vi "Autonomous Independent.vi"   [LabVIEW 2014]
doc: "This VI is called when autonomous begins, and will automatically be terminated when autonomous ends. You can carry out timed or sensor driven robot movement independently without needing to return to the caller."
uses:
  <vilib>/Rock Robotics/SystemInterfaces/i2clib/i2c_bus.ctl
  <vilib>/Rock Robotics/Network Tables/SD Read Number.vi
  <vilib>/Rock Robotics/WPI/RobotDrive/WPI_RobotDriveGetSetRefNum.vi
  <vilib>/Rock Robotics/WPI/RobotDrive/WPI_RobotDriveMecanumDrive_Cartesian.vi
  Robot Global Data.vi
panel:
  # "Be sure to right-click and choose Data Operations>>Make Current Value default if you want to save the array values with the VI"
types:
  T1 = typedef "WPI_RobotDriveDevRef.ctl" = cluster{"DevStatus":errorcluster, "Motors[]":T2[], "Square Inputs":bool, "Max Output":dbl}
  T2 = typedef "WPI_MotorControlDeviceRef.ctl" = cluster{"DeviceStatus":errorcluster, "Type":T3, "PWM":cluster{"Controller":T4, "PWM Channel":T5, "DeadBand":T6}, "CAN":cluster{"Device Number":u8, "Control Mode":T7, "Semaphore":T8, "Max Vout":dbl, "TalonSRX Control Mode":T9}, "Invert":bool, "TransformRef":T10, "InvTransformRef":T10}
  T3 = typedef "WPI_MotorControlType.ctl" = enum16{"PWM", "CAN", "CANTalonSRX"}
  T4 = typedef "FPGA_TypedefDigitalModule.ctl" = enum16{"Controller 1"}
  T5 = typedef "FPGA_DIOPWMChannel.ctl" = enum8{"PWM 0", "PWM 1", "PWM 2", "PWM 3", "PWM 4", "PWM 5", "PWM 6", "PWM 7", "PWM 8", "PWM 9", "PWM MXP 0", "PWM MXP 1", "PWM MXP 2", "PWM MXP 3", "PWM MXP 4", "PWM MXP 5", "PWM MXP 6", "PWM MXP 7", "PWM MXP 8", "PWM MXP 9", "Invalid"}
  T6 = typedef "WPI_PWMDeadband.ctl" = cluster{"Name":string, "maxPositivePwm":i32, "minPositivePwm":i32, "centerPwm":i32, "maxNegativePwm":i32, "minNegativePwm":i32, "angularRange":u16}
  T7 = typedef "WPI_CANJaguar_ControlMode.ctl" = enum8{"Percent VBus", "Current", "Speed", "Position", "Voltage"}
  T8 = typedef "Semaphore RefNum" = refnum<k1>
  T9 = typedef "WPI_CANTalonSRX_APIControlMode.ctl" = enum8{"Percent VBus", "Speed", "Position", "Slave", "Unchanged / Invalid"}
  T10 = typedef "WPI_PWMTransform_ConPane.ctl" = refnum<vi>
  T11 = typedef "WPI_EncoderDevRef.ctl" = cluster{"DevStatus":errorcluster, "EncoderIndex":T12, "CounterIndex":T13, "DistancePerCount":dbl, "Decoding Type":T14}
  T12 = typedef "FPGA_EncoderIdx.ctl" = enum8{"Enc 0", "Enc 1", "Enc 2", "Enc 3", "Enc 4", "Enc 5", "Enc 6", "Enc 7", "Invalid"}
  T13 = typedef "FPGA_CounterCtrSystemIndex.ctl" = enum8{"Ctr 0", "Ctr 1", "Ctr 2", "Ctr 3", "Ctr 4", "Ctr 5", "Ctr 6", "Ctr 7", "Invalid"}
  T14 = typedef "WPI_EncoderType.ctl" = enum16{"1x", "2x", "4x"}
  T15 = typedef "WPI_GyroDevRef.ctl" = cluster{"DevStatus":errorcluster, "Analog Module":T16, "Analog Channel":T17, "Offset":dbl, "Gain (VoltsPerDegree/Second)":dbl}
  T16 = typedef "FPGA_TypedefAnalogModule.ctl" = enum16{"Controller 1"}
  T17 = typedef "FPGA_AIChannel.ctl" = enum8{"AI 0", "AI 1", "AI 2", "AI 3", "AI MXP 0", "AI MXP 1", "AI MXP 2", "AI MXP 3", "Invalid"}
  T18 = typedef "WPI_I2CDevRef.ctl" = cluster{"DevStatus":errorcluster, "Controller":T4, "Device Address":u8, "Handle":i32, "I2C Bus":T19}
  T19 = typedef "i2c_bus.ctl" = enum16{"I2C On-Board", "I2C MXP", "Invalid"}
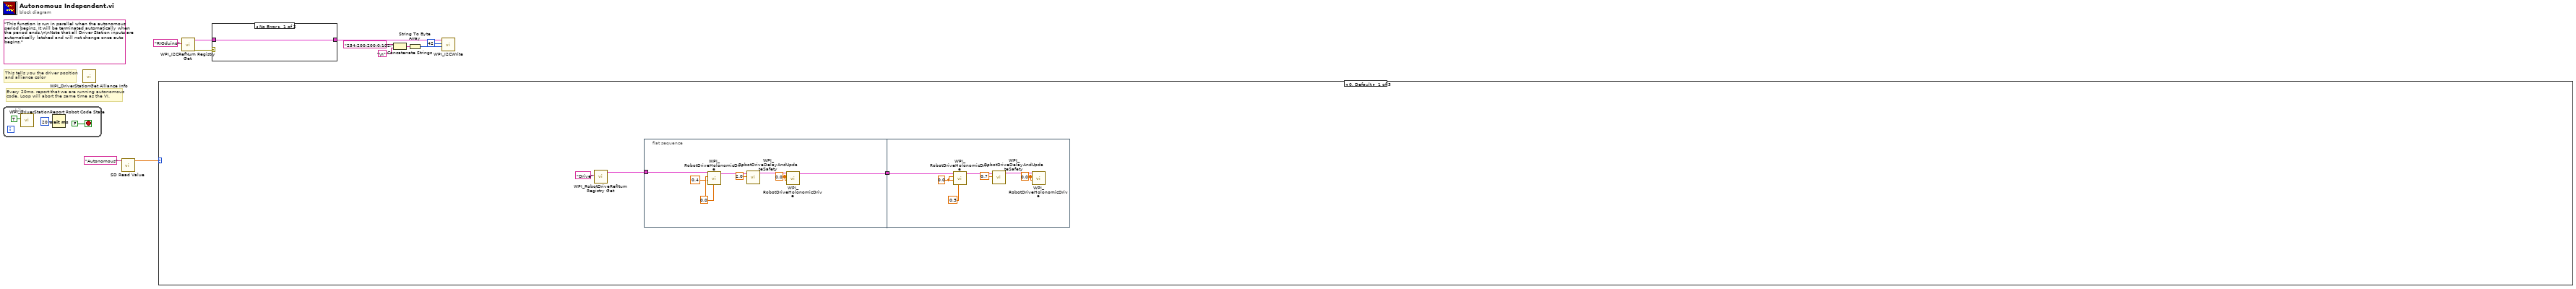
[diagram p0: block diagram]
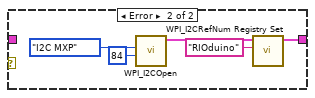
[diagram p2: hidden frame]
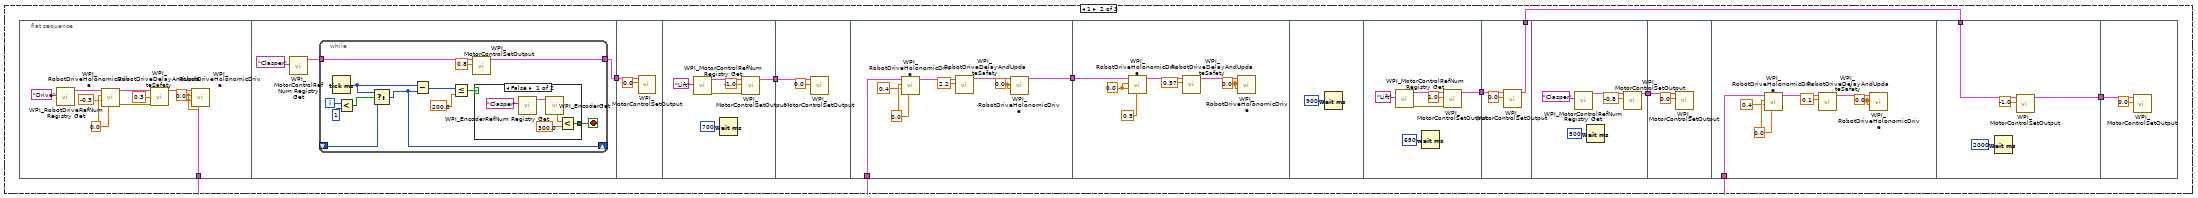
[diagram p3: hidden frame]
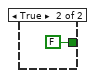
[diagram p4: hidden frame]
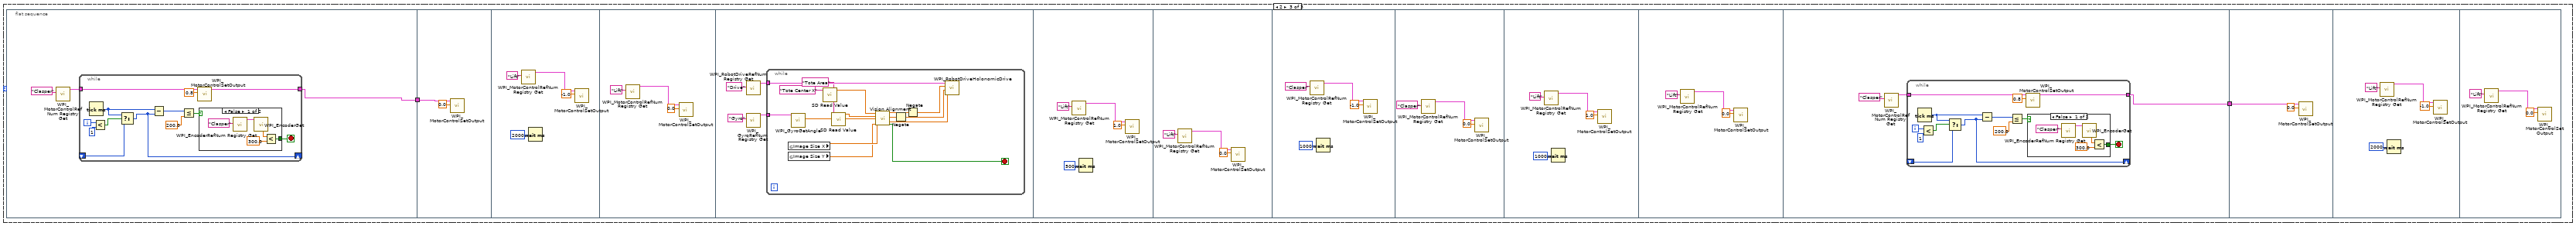
[diagram p5: hidden frame]
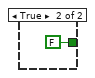
[diagram p6: hidden frame]
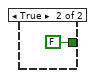
[diagram p7: hidden frame]
diagram:
  (unwired) "This function is run in parallel when the autonomous period begins. It will be terminated automatically when the period ends.\n\nNote that all Driver Station inputs are automatically latched and will not change once auto begins."
  # "Every 20ms, report that we are running autonomous\ncode. Loop will abort the same time as the VI."
  # "This tells you the driver position\nand alliance color"
  n1 = while {
    stop <- FALSE stop-if-true
    n2 = call <vilib>:"WPI_DriverStationReport Robot Code State.vi"("Autonomous"=TRUE) -> ()  [unwired: 10 in, 1 out]
    n3 = Wait (ms)(milliseconds to wait=u32 20) -> ()  [unwired: 1 out]
  }
  n4 = call <vilib>:"WPI_DriverStationGet Alliance Info.vi"() -> ()  [unwired: 12 out]
  n5 = call-poly <vilib>:"SD Read Value.vi"("Name"="Autonomous") -> ("Numeric"=w10:dbl)  [unwired: 8 in, 2 out]
  n6 = case shown="0, Default" w10 {
    frame 0, Default {
      n7 = call <vilib>:"WPI_RobotDriveRefNum Registry Get.vi"("refnum name"="Drive") -> ("RobotDriveDevRef"=w15:T1)  [unwired: 9 in, 1 out]
      n8 = flat-sequence {
        tunnel: [w19] -> w17
        tunnel: w15 -> [w18]
        tunnel: w17 -> [w26]
        frame #0 {
          w21 = 0.0
          w22 = 0.0 ("X")
          n9 = call-poly <vilib>:"WPI_RobotDriveHolonomicDrive.vi"("Rotation"=w21, "Y"=0.4 ("X"), "X"=w21, "RobotDriveDevRef"=w18) -> ("RobotDriveDevRef"=w25:T1)  [unwired: 5 in, 2 out]
          n10 = call <vilib>:"WPI_RobotDriveDelayAndUpdateSafety.vi"("Delay (s)"=2.0, "RobotDriveDevRef"=w25) -> ("RobotDriveDevRef 2"=w23:T1)  [unwired: 8 in, 1 out]
          n11 = call-poly <vilib>:"WPI_RobotDriveHolonomicDrive.vi"("Rotation"=w22, "Y"=w22, "X"=w22, "RobotDriveDevRef"=w23) -> ("RobotDriveDevRef"=w19:T1)  [unwired: 5 in, 2 out]
        }
        frame #1 {
          w30 = 0.0 ("X")
          w32 = 0.0 ("X")
          n12 = call-poly <vilib>:"WPI_RobotDriveHolonomicDrive.vi"("Rotation"=0.5, "Y"=w32, "X"=w32, "RobotDriveDevRef"=w26) -> ("RobotDriveDevRef"=w27:T1)  [unwired: 5 in, 2 out]
          n13 = call <vilib>:"WPI_RobotDriveDelayAndUpdateSafety.vi"("Delay (s)"=0.7, "RobotDriveDevRef"=w27) -> ("RobotDriveDevRef 2"=w29:T1)  [unwired: 8 in, 1 out]
          n14 = call-poly <vilib>:"WPI_RobotDriveHolonomicDrive.vi"("Rotation"=w30, "Y"=w30, "X"=w30, "RobotDriveDevRef"=w29) -> ()  [unwired: 5 in, 3 out]
        }
      }
    }
    frame 1 {
      n15 = flat-sequence {
        tunnel: [w44] -> w36
        tunnel: [w51] -> w40
        tunnel: w40 -> [w74]
        tunnel: [w75] -> w39
        tunnel: w39 -> [w82]
        tunnel: w36 -> [w89]
        tunnel: [w83] -> w35
        tunnel: w35 -> [w92]
        tunnel: [w99] -> w38
        tunnel: w38 -> [w106]
        tunnel: [w105] -> w33
        tunnel: [w108] -> w37
        tunnel: w37 -> [w113]
        tunnel: w36 -> [w115]
        tunnel: [w123] -> w34
        tunnel: w33 -> [w122]
        tunnel: w34 -> [w126]
        frame #0 {
          w42 = 0.0
          w43 = 0.0 ("X")
          n16 = call <vilib>:"WPI_RobotDriveRefNum Registry Get.vi"("refnum name"="Drive") -> ("RobotDriveDevRef"=w50:T1)  [unwired: 9 in, 1 out]
          n17 = call-poly <vilib>:"WPI_RobotDriveHolonomicDrive.vi"("Rotation"=w42, "Y"=-0.3 ("X"), "X"=w42, "RobotDriveDevRef"=w50) -> ("error out"=w48:errorcluster, "RobotDriveDevRef"=w47:T1)  [unwired: 5 in, 1 out]
          n18 = call <vilib>:"WPI_RobotDriveDelayAndUpdateSafety.vi"("error in (no error)"=w48, "Delay (s)"=0.3, "RobotDriveDevRef"=w47) -> ("RobotDriveDevRef 2"=w45:T1)  [unwired: 7 in, 1 out]
          n19 = call-poly <vilib>:"WPI_RobotDriveHolonomicDrive.vi"("Rotation"=w43, "Y"=w43, "X"=w43, "RobotDriveDevRef"=w45) -> ("RobotDriveDevRef"=w44:T1)  [unwired: 5 in, 2 out]
        }
        frame #1 {
          n20 = call <vilib>:"WPI_MotorControlRefNum Registry Get.vi"("refnum name"="Clasper") -> ("MotorControlDevRef"=w52:T2)  [unwired: 9 in, 1 out]
          n21 = while {
            tunnel: w52 -> [w66]
            tunnel: [w64] -> w51
            shift-right: [w58] -> _
            shift-left: _ -> [w59]
            i -> [w57]
            stop <- w60 stop-if-true
            n22 = Tick Count (ms)() -> (millisecond timer value=w63:u32)
            n23 = Less?(x=w57, y=1) -> (x < y?=w55:bool)
            n24 = Select(t=w63, s=w55, f=w59) -> (s? t:f=w58:u32)
            n25 = Subtract(x=w63, y=w58) -> (x-y=w62:u32)
            n26 = Less Or Equal?(x=w62, y=200.0) -> (x <= y?=w61:bool)
            n27 = call <vilib>:"WPI_MotorControlSetOutput.vi"("Output"=0.8, "MotorControlDevRef"=w66) -> ("MotorControlDevRef"=w64:T2)  [unwired: 7 in, 2 out]
            n28 = case shown="False" w61 {
              tunnel: [w67 FALSE] -> w60
              frame False {
                n29 = call <vilib>:"WPI_EncoderRefNum Registry Get.vi"("refnum name"="Clasper") -> ("EncoderDevRef"=w71:T11)  [unwired: 9 in, 1 out]
                n30 = call <vilib>:"WPI_EncoderGet.vi"("EncoderDevRef"=w71) -> ("Rate"=w68:dbl)  [unwired: 5 in, 5 out]
                n31 = Less?(x=w68, y=300.0) -> (x < y?=w67:bool)
              }
              frame True {
              }
            }
          }
        }
        frame #2 {
          n32 = call <vilib>:"WPI_MotorControlSetOutput.vi"("Output"=0.0, "MotorControlDevRef"=w74) -> ()  [unwired: 7 in, 3 out]
        }
        frame #3 {
          n33 = call <vilib>:"WPI_MotorControlRefNum Registry Get.vi"("refnum name"="Lift") -> ("error out"=w79:errorcluster, "MotorControlDevRef"=w78:T2)  [unwired: 9 in]
          n34 = Wait (ms)(milliseconds to wait=u32 700) -> ()  [unwired: 1 out]
          n35 = call <vilib>:"WPI_MotorControlSetOutput.vi"("error in (no error)"=w79, "Output"=-1.0, "MotorControlDevRef"=w78) -> ("MotorControlDevRef"=w75:T2)  [unwired: 6 in, 2 out]
        }
        frame #4 {
          n36 = call <vilib>:"WPI_MotorControlSetOutput.vi"("Output"=0.0, "MotorControlDevRef"=w82) -> ()  [unwired: 7 in, 3 out]
        }
        frame #5 {
          w85 = 0.0
          w86 = 0.0 ("X")
          n37 = call-poly <vilib>:"WPI_RobotDriveHolonomicDrive.vi"("Rotation"=w85, "Y"=0.4 ("X"), "X"=w85, "RobotDriveDevRef"=w89) -> ("RobotDriveDevRef"=w90:T1)  [unwired: 5 in, 2 out]
          n38 = call <vilib>:"WPI_RobotDriveDelayAndUpdateSafety.vi"("Delay (s)"=2.2, "RobotDriveDevRef"=w90) -> ("RobotDriveDevRef 2"=w87:T1)  [unwired: 8 in, 1 out]
          n39 = call-poly <vilib>:"WPI_RobotDriveHolonomicDrive.vi"("Rotation"=w86, "Y"=w86, "X"=w86, "RobotDriveDevRef"=w87) -> ("RobotDriveDevRef"=w83:T1)  [unwired: 5 in, 2 out]
        }
        frame #6 {
          w94 = 0.0 ("X")
          w91 = 0.0 ("X")
          n40 = call-poly <vilib>:"WPI_RobotDriveHolonomicDrive.vi"("Rotation"=0.5, "Y"=w91, "X"=w91, "RobotDriveDevRef"=w92) -> ("RobotDriveDevRef"=w97:T1)  [unwired: 5 in, 2 out]
          n41 = call <vilib>:"WPI_RobotDriveDelayAndUpdateSafety.vi"("Delay (s)"=0.57, "RobotDriveDevRef"=w97) -> ("RobotDriveDevRef 2"=w95:T1)  [unwired: 8 in, 1 out]
          n42 = call-poly <vilib>:"WPI_RobotDriveHolonomicDrive.vi"("Rotation"=w94, "Y"=w94, "X"=w94, "RobotDriveDevRef"=w95) -> ()  [unwired: 5 in, 3 out]
        }
        frame #7 {
          n43 = Wait (ms)(milliseconds to wait=u32 900) -> ()  [unwired: 1 out]
        }
        frame #8 {
          n44 = call <vilib>:"WPI_MotorControlRefNum Registry Get.vi"("refnum name"="Lift") -> ("error out"=w103:errorcluster, "MotorControlDevRef"=w102:T2)  [unwired: 9 in]
          n45 = Wait (ms)(milliseconds to wait=u32 650) -> ()  [unwired: 1 out]
          n46 = call <vilib>:"WPI_MotorControlSetOutput.vi"("error in (no error)"=w103, "Output"=1.0, "MotorControlDevRef"=w102) -> ("MotorControlDevRef"=w99:T2)  [unwired: 6 in, 2 out]
        }
        frame #9 {
          n47 = call <vilib>:"WPI_MotorControlSetOutput.vi"("Output"=0.0, "MotorControlDevRef"=w106) -> ("MotorControlDevRef"=w105:T2)  [unwired: 7 in, 2 out]
        }
        frame #10 {
          n48 = call <vilib>:"WPI_MotorControlRefNum Registry Get.vi"("refnum name"="Clasper") -> ("MotorControlDevRef"=w110:T2)  [unwired: 9 in, 1 out]
          n49 = Wait (ms)(milliseconds to wait=u32 500) -> ()  [unwired: 1 out]
          n50 = call <vilib>:"WPI_MotorControlSetOutput.vi"("Output"=-0.8, "MotorControlDevRef"=w110) -> ("MotorControlDevRef"=w108:T2)  [unwired: 7 in, 2 out]
        }
        frame #11 {
          n51 = call <vilib>:"WPI_MotorControlSetOutput.vi"("Output"=0.0, "MotorControlDevRef"=w113) -> ()  [unwired: 7 in, 3 out]
        }
        frame #12 {
          w117 = 0.0
          w118 = 0.0 ("X")
          n52 = call-poly <vilib>:"WPI_RobotDriveHolonomicDrive.vi"("Rotation"=w117, "Y"=0.4 ("X"), "X"=w117, "RobotDriveDevRef"=w115) -> ("RobotDriveDevRef"=w121:T1)  [unwired: 5 in, 2 out]
          n53 = call <vilib>:"WPI_RobotDriveDelayAndUpdateSafety.vi"("Delay (s)"=0.1, "RobotDriveDevRef"=w121) -> ("RobotDriveDevRef 2"=w119:T1)  [unwired: 8 in, 1 out]
          n54 = call-poly <vilib>:"WPI_RobotDriveHolonomicDrive.vi"("Rotation"=w118, "Y"=w118, "X"=w118, "RobotDriveDevRef"=w119) -> ()  [unwired: 5 in, 3 out]
        }
        frame #13 {
          n55 = Wait (ms)(milliseconds to wait=u32 2000) -> ()  [unwired: 1 out]
          n56 = call <vilib>:"WPI_MotorControlSetOutput.vi"("Output"=-1.0, "MotorControlDevRef"=w122) -> ("MotorControlDevRef"=w123:T2)  [unwired: 7 in, 2 out]
        }
        frame #14 {
          n57 = call <vilib>:"WPI_MotorControlSetOutput.vi"("Output"=0.0, "MotorControlDevRef"=w126) -> ()  [unwired: 7 in, 3 out]
        }
      }
    }
    frame 2 {
      n58 = flat-sequence {
        tunnel: [w130] -> w128
        tunnel: w128 -> [w152]
        tunnel: [w203] -> w129
        tunnel: w129 -> [w224]
        frame #0 {
          n59 = call <vilib>:"WPI_MotorControlRefNum Registry Get.vi"("refnum name"="Clasper") -> ("MotorControlDevRef"=w131:T2)  [unwired: 9 in, 1 out]
          n60 = while {
            tunnel: w131 -> [w145]
            tunnel: [w143] -> w130
            shift-right: [w137] -> _
            shift-left: _ -> [w138]
            i -> [w136]
            stop <- w139 stop-if-true
            n61 = Tick Count (ms)() -> (millisecond timer value=w142:u32)
            n62 = Less?(x=w136, y=1) -> (x < y?=w134:bool)
            n63 = Select(t=w142, s=w134, f=w138) -> (s? t:f=w137:u32)
            n64 = Subtract(x=w142, y=w137) -> (x-y=w141:u32)
            n65 = Less Or Equal?(x=w141, y=200.0) -> (x <= y?=w140:bool)
            n66 = call <vilib>:"WPI_MotorControlSetOutput.vi"("Output"=0.8, "MotorControlDevRef"=w145) -> ("MotorControlDevRef"=w143:T2)  [unwired: 7 in, 2 out]
            n67 = case shown="False" w140 {
              tunnel: [w146 FALSE] -> w139
              frame False {
                n68 = call <vilib>:"WPI_EncoderRefNum Registry Get.vi"("refnum name"="Clasper") -> ("EncoderDevRef"=w150:T11)  [unwired: 9 in, 1 out]
                n69 = call <vilib>:"WPI_EncoderGet.vi"("EncoderDevRef"=w150) -> ("Rate"=w147:dbl)  [unwired: 5 in, 5 out]
                n70 = Less?(x=w147, y=300.0) -> (x < y?=w146:bool)
              }
              frame True {
              }
            }
          }
        }
        frame #1 {
          n71 = call <vilib>:"WPI_MotorControlSetOutput.vi"("Output"=0.0, "MotorControlDevRef"=w152) -> ()  [unwired: 7 in, 3 out]
        }
        frame #2 {
          n72 = call <vilib>:"WPI_MotorControlRefNum Registry Get.vi"("refnum name"="Lift") -> ("MotorControlDevRef"=w156:T2)  [unwired: 9 in, 1 out]
          n73 = Wait (ms)(milliseconds to wait=u32 2000) -> ()  [unwired: 1 out]
          n74 = call <vilib>:"WPI_MotorControlSetOutput.vi"("Output"=-1.0, "MotorControlDevRef"=w156) -> ()  [unwired: 7 in, 3 out]
        }
        frame #3 {
          n75 = call <vilib>:"WPI_MotorControlRefNum Registry Get.vi"("refnum name"="Lift") -> ("MotorControlDevRef"=w159:T2)  [unwired: 9 in, 1 out]
          n76 = call <vilib>:"WPI_MotorControlSetOutput.vi"("Output"=0.0, "MotorControlDevRef"=w159) -> ()  [unwired: 7 in, 3 out]
        }
        frame #4 {
          n77 = call <vilib>:"WPI_RobotDriveRefNum Registry Get.vi"("refnum name"="Drive") -> ("RobotDriveDevRef"=w163:T1)  [unwired: 9 in, 1 out]
          n78 = call <vilib>:"WPI_GyroRefNum Registry Get.vi"("refnum name"="Gyro") -> ("GyroDevRef"=w162:T15)  [unwired: 9 in, 1 out]
          n79 = while {
            tunnel: w163 -> [w179]
            tunnel: w162 -> [w176]
            stop <- w165 stop-if-true
            n80 = global read "Robot Global Data.vi" "Image Size X"() -> (w178:dbl)
            n81 = global read "Robot Global Data.vi" "Image Size Y"() -> (w177:dbl)
            n82 = call <vilib>:"WPI_GyroGetAngle.vi"("GyroDevRef"=w176) -> ("Angle"=w175:dbl)  [unwired: 7 in, 3 out]
            n83 = call-poly <vilib>:"SD Read Value.vi"("Name"="Tote Center X") -> ("Numeric"=w170:dbl)  [unwired: 8 in, 2 out]
            n84 = call-poly <vilib>:"SD Read Value.vi"("Name"="Tote Area") -> ("Numeric"=w169:dbl)  [unwired: 8 in, 2 out]
            n85 = call "Vision Alignment.vi"("Center of Mass X"=w170, "Area"=w169, "Gyro Angle"=w175, "Res X"=w178, "Res Y"=w177) -> ("Mecanum X Output"=w174:dbl, "Mecanum Y Output"=w173:dbl, "Rotation Output"=w172:dbl, "At tote?"=w165:bool)  [unwired: 7 in]
            n86 = Negate(x=w173) -> (-x=w166:dbl)
            n87 = Negate(x=w174) -> (-x=w167:dbl)
            n88 = call-poly <vilib>:"WPI_RobotDriveHolonomicDrive.vi"("Rotation"=w172, "Y"=w166, "X"=w167, "RobotDriveDevRef"=w179) -> ()  [unwired: 5 in, 3 out]
          }
        }
        frame #5 {
          n89 = call <vilib>:"WPI_MotorControlRefNum Registry Get.vi"("refnum name"="Lift") -> ("MotorControlDevRef"=w182:T2)  [unwired: 9 in, 1 out]
          n90 = Wait (ms)(milliseconds to wait=u32 500) -> ()  [unwired: 1 out]
          n91 = call <vilib>:"WPI_MotorControlSetOutput.vi"("Output"=1.0, "MotorControlDevRef"=w182) -> ()  [unwired: 7 in, 3 out]
        }
        frame #6 {
          n92 = call <vilib>:"WPI_MotorControlRefNum Registry Get.vi"("refnum name"="Lift") -> ("MotorControlDevRef"=w185:T2)  [unwired: 9 in, 1 out]
          n93 = call <vilib>:"WPI_MotorControlSetOutput.vi"("Output"=0.0, "MotorControlDevRef"=w185) -> ()  [unwired: 7 in, 3 out]
        }
        frame #7 {
          n94 = call <vilib>:"WPI_MotorControlRefNum Registry Get.vi"("refnum name"="Clasper") -> ("MotorControlDevRef"=w189:T2)  [unwired: 9 in, 1 out]
          n95 = Wait (ms)(milliseconds to wait=u32 1000) -> ()  [unwired: 1 out]
          n96 = call <vilib>:"WPI_MotorControlSetOutput.vi"("Output"=-1.0, "MotorControlDevRef"=w189) -> ()  [unwired: 7 in, 3 out]
        }
        frame #8 {
          n97 = call <vilib>:"WPI_MotorControlRefNum Registry Get.vi"("refnum name"="Clasper") -> ("MotorControlDevRef"=w192:T2)  [unwired: 9 in, 1 out]
          n98 = call <vilib>:"WPI_MotorControlSetOutput.vi"("Output"=0.0, "MotorControlDevRef"=w192) -> ()  [unwired: 7 in, 3 out]
        }
        frame #9 {
          n99 = call <vilib>:"WPI_MotorControlRefNum Registry Get.vi"("refnum name"="Lift") -> ("MotorControlDevRef"=w196:T2)  [unwired: 9 in, 1 out]
          n100 = Wait (ms)(milliseconds to wait=u32 1000) -> ()  [unwired: 1 out]
          n101 = call <vilib>:"WPI_MotorControlSetOutput.vi"("Output"=1.0, "MotorControlDevRef"=w196) -> ()  [unwired: 7 in, 3 out]
        }
        frame #10 {
          n102 = call <vilib>:"WPI_MotorControlRefNum Registry Get.vi"("refnum name"="Lift") -> ("MotorControlDevRef"=w199:T2)  [unwired: 9 in, 1 out]
          n103 = call <vilib>:"WPI_MotorControlSetOutput.vi"("Output"=0.0, "MotorControlDevRef"=w199) -> ()  [unwired: 7 in, 3 out]
        }
        frame #11 {
          n104 = call <vilib>:"WPI_MotorControlRefNum Registry Get.vi"("refnum name"="Clasper") -> ("MotorControlDevRef"=w201:T2)  [unwired: 9 in, 1 out]
          n105 = while {
            tunnel: w201 -> [w216]
            tunnel: [w214] -> w203
            shift-right: [w208] -> _
            shift-left: _ -> [w209]
            i -> [w207]
            stop <- w210 stop-if-true
            n106 = Tick Count (ms)() -> (millisecond timer value=w213:u32)
            n107 = Less?(x=w207, y=1) -> (x < y?=w205:bool)
            n108 = Select(t=w213, s=w205, f=w209) -> (s? t:f=w208:u32)
            n109 = Subtract(x=w213, y=w208) -> (x-y=w212:u32)
            n110 = Less Or Equal?(x=w212, y=200.0) -> (x <= y?=w211:bool)
            n111 = call <vilib>:"WPI_MotorControlSetOutput.vi"("Output"=0.8, "MotorControlDevRef"=w216) -> ("MotorControlDevRef"=w214:T2)  [unwired: 7 in, 2 out]
            n112 = case shown="False" w211 {
              tunnel: [w217 FALSE] -> w210
              frame False {
                n113 = call <vilib>:"WPI_EncoderRefNum Registry Get.vi"("refnum name"="Clasper") -> ("EncoderDevRef"=w221:T11)  [unwired: 9 in, 1 out]
                n114 = call <vilib>:"WPI_EncoderGet.vi"("EncoderDevRef"=w221) -> ("Rate"=w218:dbl)  [unwired: 5 in, 5 out]
                n115 = Less?(x=w218, y=300.0) -> (x < y?=w217:bool)
              }
              frame True {
              }
            }
          }
        }
        frame #12 {
          n116 = call <vilib>:"WPI_MotorControlSetOutput.vi"("Output"=0.0, "MotorControlDevRef"=w224) -> ()  [unwired: 7 in, 3 out]
        }
        frame #13 {
          n117 = call <vilib>:"WPI_MotorControlRefNum Registry Get.vi"("refnum name"="Lift") -> ("MotorControlDevRef"=w227:T2)  [unwired: 9 in, 1 out]
          n118 = Wait (ms)(milliseconds to wait=u32 2000) -> ()  [unwired: 1 out]
          n119 = call <vilib>:"WPI_MotorControlSetOutput.vi"("Output"=-1.0, "MotorControlDevRef"=w227) -> ()  [unwired: 7 in, 3 out]
        }
        frame #14 {
          n120 = call <vilib>:"WPI_MotorControlRefNum Registry Get.vi"("refnum name"="Lift") -> ("MotorControlDevRef"=w230:T2)  [unwired: 9 in, 1 out]
          n121 = call <vilib>:"WPI_MotorControlSetOutput.vi"("Output"=0.0, "MotorControlDevRef"=w230) -> ()  [unwired: 7 in, 3 out]
        }
      }
    }
  }
  n122 = call <vilib>:"WPI_I2CRefNum Registry Get.vi"("refnum name"="RIOduino") -> ("error out"=w6:errorcluster, "I2CDevRef"=w5:T18)  [unwired: 9 in]
  n123 = case shown="No Error" w6 {
    tunnel: w5 -> [w232 _]
    tunnel: [w232 w233] -> w4
    frame No Error {
    }
    frame Error {
      n124 = call <vilib>:"WPI_I2COpen.vi"("Device Address"=u8 84, "I2C Bus"=i2c_bus."I2C MXP") -> ("I2CDevRef"=w237:T18)  [unwired: 8 in, 1 out]
      n125 = call <vilib>:"WPI_I2CRefNum Registry Set.vi"("refnum name"="RIOduino", "I2CDevRef"=w237) -> ("I2CDevRef"=w233:T18)  [unwired: 8 in, 1 out]
    }
  }
  n126 = Concatenate Strings("254;200;200;0;102;" ("string"), "\n") -> (w3:string)
  n127 = String To Byte Array(string=w3) -> (unsigned byte array=w7:u8[])
  n128 = call <vilib>:"WPI_I2CWrite.vi"("I2CDataToSend"=w7, "I2CRegister"=u8 42, "I2CDevRef"=w4) -> ()  [unwired: 7 in, 2 out]
